vi "Create.vi"(8 "error in (no error)":errorcluster, 9 "Delta value":refnum<class "Data.lvclass">, 10 "Ending":refnum<class "Data.lvclass">, 11 "Begin":refnum<class "Data.lvclass">) -> (0 "error out":errorcluster, 3 "Range out":refnum<class "Range.lvclass">)   [LabVIEW 2012, in "MDSplus.lvlib" / "Range.lvclass"]
uses:
  <vilib>/MDSplus/Classes/Data_Class/Compound_Class/Range_Class/Range.lvclass
  <vilib>/MDSplus/Classes/Data_Class/Data.lvclass
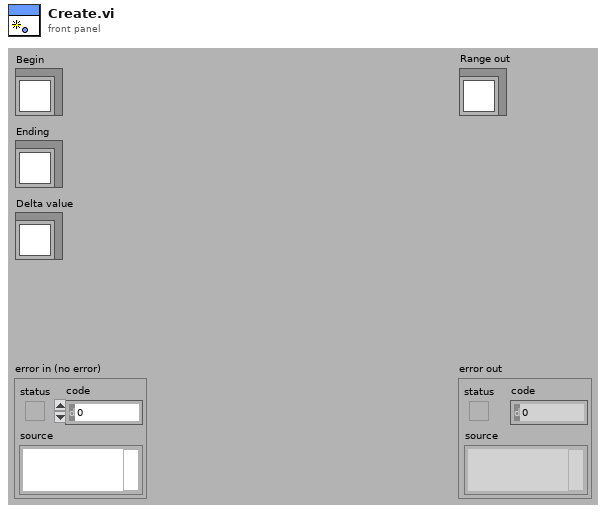
[diagram p1: front panel]
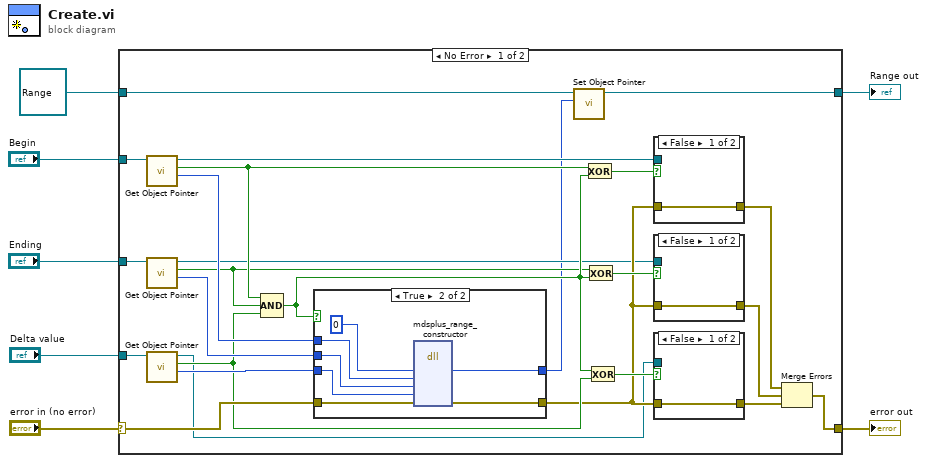
[diagram p0: block diagram]
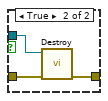
[diagram p2: hidden frame]
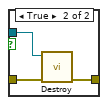
[diagram p3: hidden frame]
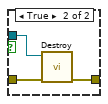
[diagram p4: hidden frame]
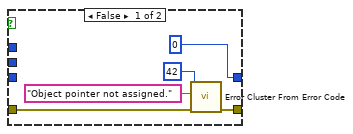
[diagram p5: hidden frame]
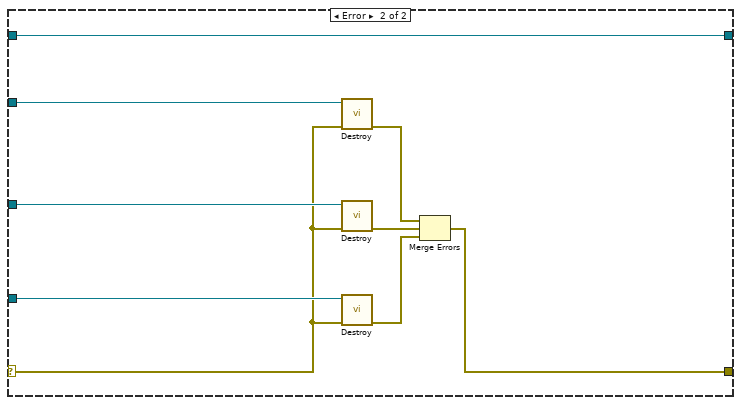
[diagram p6: hidden frame]
diagram:
  n1 = case shown="No Error" "error in (no error)" {
    selector: "error in (no error)" -> [w26 w58]
    tunnel: [w11 w57] -> w6
    tunnel: [w9 w65] -> w4
    tunnel: refnum<class "Range.lvclass"> refnum ("Range in") -> [w10 w65]
    tunnel: "Begin" -> [w32 w64]
    tunnel: "Ending" -> [w31 w63]
    tunnel: "Delta value" -> [w30 w62]
    frame No Error {
      n2 = call-dynamic "Get Object Pointer.vi"("Data in"=w32) -> ("Object Pointer"=w27:i64, "Assigned object pointer?"=w22:bool, "Data out"=w17:refnum<class "Data.lvclass">)  [unwired: 8 in]
      n3 = call-dynamic "Get Object Pointer.vi"("Data in"=w31) -> ("Object Pointer"=w28:i64, "Assigned object pointer?"=w19:bool, "Data out"=w16:refnum<class "Data.lvclass">)  [unwired: 8 in]
      n4 = call-dynamic "Get Object Pointer.vi"("Data in"=w30) -> ("Object Pointer"=w29:i64, "Assigned object pointer?"=w21:bool, "Data out"=w15:refnum<class "Data.lvclass">)  [unwired: 8 in]
      n5 = Compound Arithmetic op=AND(w22, w19, w21) -> (w20:bool)
      n6 = case shown="True" w20 {
        tunnel: w29 -> [_ w55]
        tunnel: w28 -> [_ w54]
        tunnel: w27 -> [_ w53]
        tunnel: w26 -> [w47 w52]
        tunnel: [w46 w51] -> w18
        tunnel: [i64 0 ("lvRangePtr") w50] -> w8
        frame False {
          n7 = call <vilib>:"Error Cluster From Error Code.vi"("error in (no error)"=w47, "error message (\"\")"="Object pointer not assigned." ("error message (\"\")"), "error code (0)"=42) -> ("error out"=w46:errorcluster)  [unwired: 6 in]
        }
        frame True {
          n8 = dll-call lib="MDSobjectsLVShr" fn="mdsplus_range_constructor"("lvRangePtr"=i64 0, "lvBeginDataPtrIn"=w53, "lvEndingDataPtrIn"=w54, "lvDeltaValDataPtrIn"=w55, "error"=w52) -> ("lvRangePtr"=w50:i64, "error"=w51:errorcluster)  [unwired: 7 in, 2 out]
        }
      }
      n9 = call-dynamic "Set Object Pointer.vi"("Object Pointer"=w8, "Data in"=w10) -> ("Data out"=w9:refnum<class "Range.lvclass">)  [unwired: 9 in]
      n10 = Exclusive Or(1:w20, 2:w22) -> (0:w25:bool)
      n11 = Exclusive Or(1:w20, 2:w19) -> (0:w24:bool)
      n12 = Exclusive Or(1:w21, 2:w20) -> (0:w23:bool)
      n13 = case shown="False" w25 {
        tunnel: w18 -> [w37 w40]
        tunnel: w17 -> [_ w39]
        tunnel: [w37 w38] -> w12
        frame False {
        }
        frame True {
          n14 = call-dynamic "Destroy.vi"("error in (no error)"=w40, "Data in"=w39) -> ("error out"=w38:errorcluster)  [unwired: 9 in]
        }
      }
      n15 = case shown="False" w24 {
        tunnel: w18 -> [w41 w44]
        tunnel: w16 -> [_ w43]
        tunnel: [w41 w42] -> w13
        frame False {
        }
        frame True {
          n16 = call-dynamic "Destroy.vi"("error in (no error)"=w44, "Data in"=w43) -> ("error out"=w42:errorcluster)  [unwired: 9 in]
        }
      }
      n17 = case shown="False" w23 {
        tunnel: w18 -> [w33 w36]
        tunnel: w15 -> [_ w35]
        tunnel: [w33 w34] -> w14
        frame False {
        }
        frame True {
          n18 = call-dynamic "Destroy.vi"("error in (no error)"=w36, "Data in"=w35) -> ("error out"=w34:errorcluster)  [unwired: 9 in]
        }
      }
      n19 = Merge Errors(w12, w13, w14) -> (w11:errorcluster)
    }
    frame Error {
      n20 = call-dynamic "Destroy.vi"("error in (no error)"=w58, "Data in"=w64) -> ("error out"=w59:errorcluster)  [unwired: 9 in]
      n21 = call-dynamic "Destroy.vi"("error in (no error)"=w58, "Data in"=w63) -> ("error out"=w61:errorcluster)  [unwired: 9 in]
      n22 = call-dynamic "Destroy.vi"("error in (no error)"=w58, "Data in"=w62) -> ("error out"=w60:errorcluster)  [unwired: 9 in]
      n23 = Merge Errors(w59, w61, w60) -> (w57:errorcluster)
    }
  }
  "error out" <- w6
  "Range out" <- w4
